vi "UseThisProgramFinal_AlexV1 simulated input.vi"() -> ()   [LabVIEW 2012]
uses:
  <vilib>/measure/mamon.llb/Trigger Detection for N Channel.vi
  <vilib>/express/express analysis/Spectral/Block/exnSpectralBlock spectral measurements RMS poly.vi
  <vilib>/express/express analysis/Spectral/Block/exnSpectralBlock spectral measurements RMS DDT.vi
  <vilib>/express/express analysis/Spectral/XNode/ExpressSpectralMeasurementsBlockNode.xnode
  <vilib>/measure/NI_MAPro.lvlib
panel:
  in  "play shifted audio":bool
  in  "autotune on?":bool
  in  "manual frequency \nselection":dbl
  in  "modulation frequency":dbl=3.0 caption="Frequency"
  in  "modulation amplitude":dbl=1.0 caption="Amplitude"
  in  "trigger level":dbl[](array[numeric]) format="%0.2f"
  in  "simulated frequency":dbl=700.0 caption="Frequency"
  out "Frequency Played":dbl
  out "FFT Original":waveform(dbl)(graph)
  out "Frequency Off By":dbl
  out "Output Frequency":dbl
  out "Note Closest To":string
  out "Shifted Waveform":waveform(dbl)(graph)
  out "Original Waveform":dynamicdata(graph)
  # "yea"
  # "nay"
  # "detect when pluck string, add digital effects, analog switch/potentiometer, playing a song would be awesome"
  # "nay"
  # "yea"
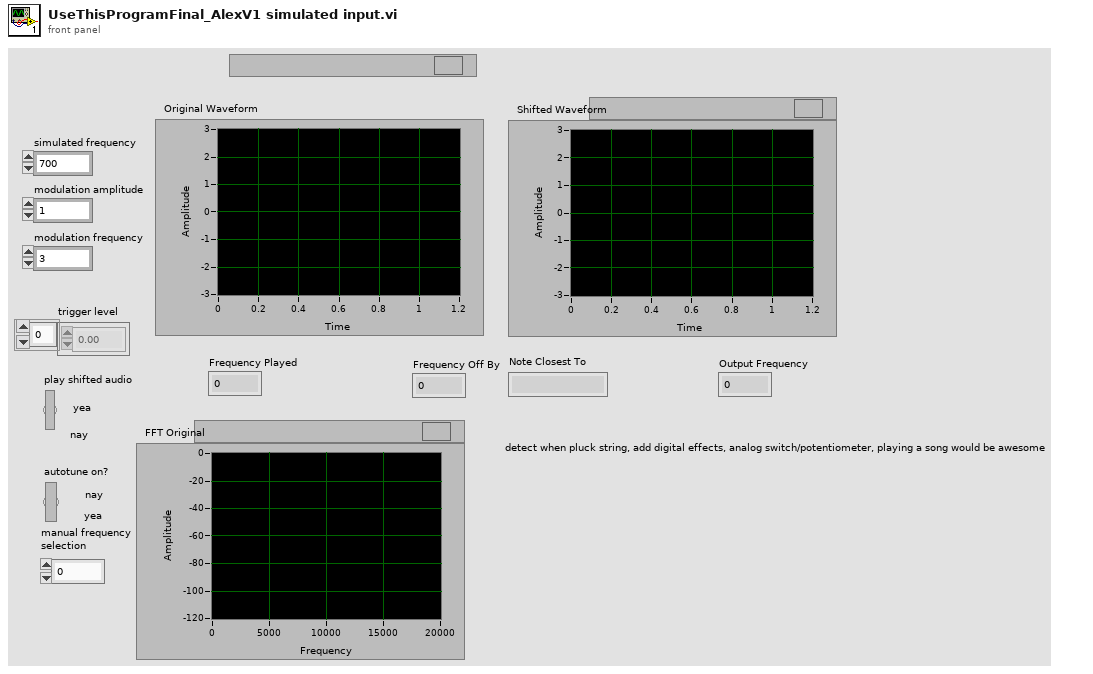
[diagram p1: front panel]
types:
  T1 = cluster{"averaging mode":u16, "weighting mode":u16, "number of averages":u32}
  T2 = cluster{"dB On (F)":bool, "unwrap phase (F)":bool, "convert to degree (F)":bool}
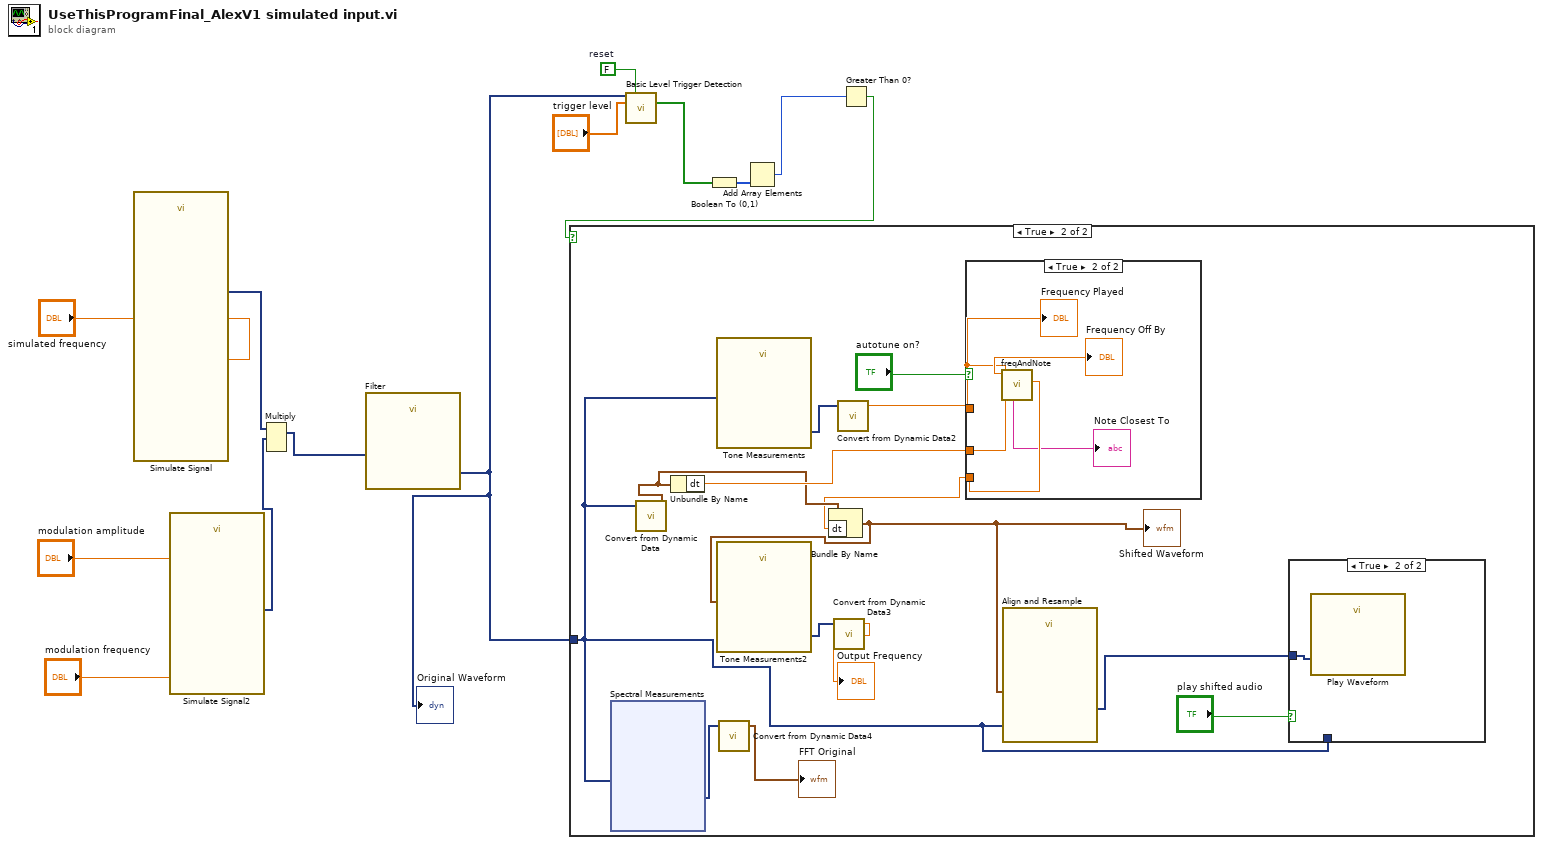
[diagram p0: block diagram]
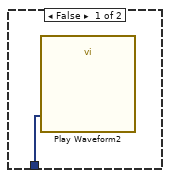
[diagram p3: hidden frame]
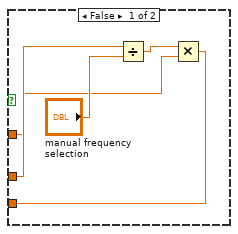
[diagram p4: hidden frame]
diagram:
  w8 = FALSE  # reset
  n1 = call "Simulate Signal"("Frequency"="simulated frequency") -> ("Sine with Uniform Noise"=w13:dynamicdata)  [unwired: 13 in, 1 out]
  n2 = call "Simulate Signal2"("Frequency"="modulation frequency", "Amplitude"="modulation amplitude") -> ("Sine"=w12:dynamicdata)  [unwired: 12 in, 1 out]
  n3 = Multiply(1:w12, 2:w13) -> (0:w11:dynamicdata)  [unwired: 1 in, 1 out]
  n4 = call "Filter"("Signal"=w11) -> ("Filtered Signal"=w1:dynamicdata)  [unwired: 9 in, 1 out]
  "Original Waveform" <- w1
  n5 = call-poly <vilib>:"Basic Level Trigger Detection.vi"("signal in"=w1, "reset"=w8, "level"="trigger level") -> ("trigger detected?"=w5:bool[])  [unwired: 10 in, 2 out]
  n6 = Boolean To (0,1)(Boolean=w5) -> (0, 1=w3:i16[])
  n7 = Add Array Elements(numeric array=w3) -> (sum=w2:i16)
  n8 = Greater Than 0?(x=w2) -> (x > 0?=w4:bool)
  n9 = case shown="True" w4 {
    tunnel: w1 -> [_ w15]
    frame False {
    }
    frame True {
      n10 = xnode "Spectral Measurements"("Signals"=w15) -> ("FFT - (RMS)"=w23:dynamicdata)  [unwired: 1 in, 2 out]
      n11 = call "Convert from Dynamic Data"("Dynamic Data Type"=w15) -> ("Waveform"=w21:waveform(dbl))  [unwired: 3 in]
      n12 = Unbundle By Name(w21) -> ("dt"=w27:dbl)
      n13 = call "Tone Measurements"("Signals"=w15) -> ("Frequency"=w26:dynamicdata)  [unwired: 8 in, 2 out]
      n14 = call "Convert from Dynamic Data4"("Dynamic Data Type"=w23) -> ("Waveform"=→"FFT Original":waveform(dbl))  [unwired: 3 in]
      n15 = call "Convert from Dynamic Data2"("Dynamic Data Type"=w26) -> ("Scalar"=w19:dbl)  [unwired: 3 in]
      n16 = case shown="True" "autotune on?" {
        tunnel: w27 -> [w34 w39]
        tunnel: [w30 w38] -> w18
        tunnel: w19 -> [w32 w35]
        frame False {
          n17 = Divide(x=w34, y="manual frequency \nselection") -> (x/y=w31:dbl)
          n18 = Multiply(x=w31, y=w32) -> (x*y=w30:dbl)
        }
        frame True {
          n19 = call "freqAndNote.vi"("dt Original"=w39, "Frequency In"=w35) -> ("output dt"=w38:dbl, "Frequency Off"=→"Frequency Off By":dbl, "Note Closest To"=→"Note Closest To":string)  [unwired: 6 in, 1 out]
          "Frequency Played" <- w35
        }
      }
      n20 = Bundle By Name(cluster=w21, "dt"=w18) -> (w20:waveform(dbl))
      "Shifted Waveform" <- w20
      n21 = call "Tone Measurements2"("Signals"=w20) -> ("Frequency"=w25:dynamicdata)  [unwired: 8 in, 2 out]
      n22 = call "Convert from Dynamic Data3"("Dynamic Data Type"=w25) -> ("Scalar"=→"Output Frequency":dbl)  [unwired: 3 in]
      n23 = call "Align and Resample"("Reference Signal"=w15, "Signals"=w20) -> ("Resampled Signals"=w14:dynamicdata)  [unwired: 7 in, 2 out]
      n24 = case shown="True" "play shifted audio" {
        tunnel: w14 -> [_ w29]
        tunnel: w15 -> [w28 _]
        frame False {
          n25 = call "Play Waveform2"("Data"=w28) -> ()  [unwired: 18 in, 1 out]
        }
        frame True {
          n26 = call "Play Waveform"("Data"=w29) -> ()  [unwired: 18 in, 1 out]
        }
      }
    }
  }
